vi "ValidateWSDL.vi"(8 "error in (no error)":errorcluster, 11 "WSDL URL":string) -> (0 "error out":errorcluster, 3 "WSDL URL (out)":string)   [LabVIEW 2017, in "WebServiceImporter.lvlib" / "ProxyDll Generator.lvlib"]
doc: "Download WSDL from given URL, validate WSDL content, ..."
uses:
  <vilib>/Platform/WebService/ProxyDll Generator/ProxyDll Generator.lvlib
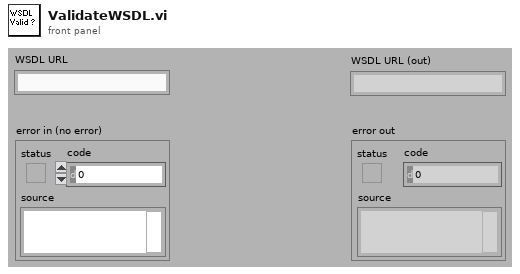
[diagram p1: front panel]
types:
  T1 = cluster{"Need Proxy":bool, "Username":string, "Password":string, "Domain":string, "Address":string, "Port":i32, "Need Authentication":bool}
  T2 = cluster{"Need Authentication":bool, "Username":string, "Password":string, "Domain":string}
  T3 = cluster{"Use Proxy Server":bool, "Address":string, "Port":u32}
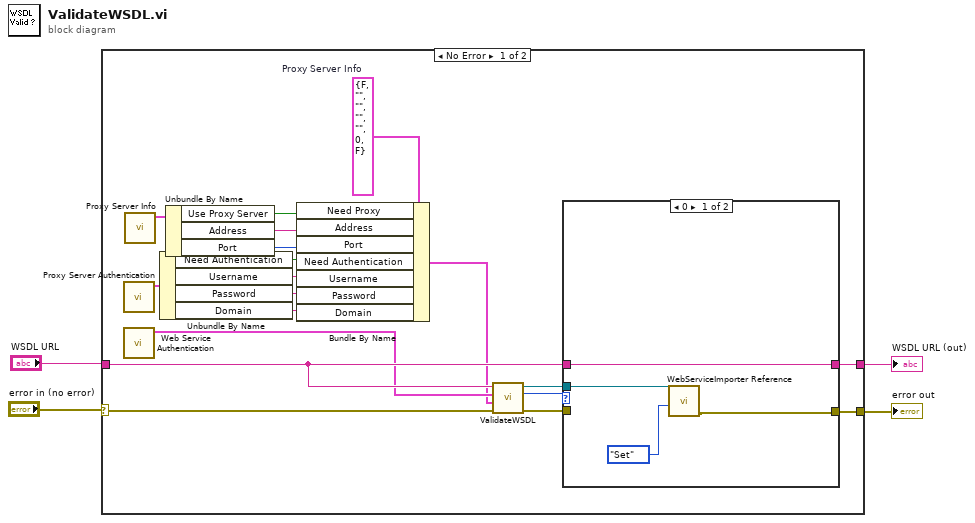
[diagram p0: block diagram]
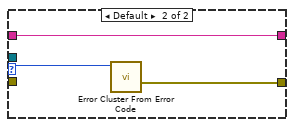
[diagram p2: hidden frame]
diagram:
  n1 = case shown="No Error" "error in (no error)" {
    selector: "error in (no error)" -> [w23 w32]
    tunnel: [w21 w32] -> w4
    tunnel: "WSDL URL" -> [w20 w31]
    tunnel: [w19 w31] -> w1
    frame No Error {
      w6 = T1 {"Need Proxy"=FALSE, "Username"="", "Password"="", "Domain"="", "Address"="", "Port"=0, "Need Authentication"=FALSE}  # Proxy Server Info
      n2 = call <vilib>:"Proxy Server Authentication.vi"() -> ("Web Service Authentication 2"=w11:T2)  [unwired: 10 in, 1 out]
      n3 = call <vilib>:"Web Service Authentication.vi"() -> ("Web Service Authentication 2"=w16:T2)  [unwired: 10 in, 1 out]
      n4 = call <vilib>:"Proxy Server Info.vi"() -> ("Proxy Server Info 2"=w15:T3)  [unwired: 10 in, 1 out]
      n5 = Unbundle By Name(w11) -> ("Need Authentication"=w10:bool, "Username"=w9:string, "Password"=w8:string, "Domain"=w7:string)
      n6 = Unbundle By Name(w15) -> ("Use Proxy Server"=w14:bool, "Address"=w13:string, "Port"=w12:u32)
      n7 = Bundle By Name(cluster=w6, "Need Proxy"=w14, "Address"=w13, "Port"=w12, "Need Authentication"=w10, "Username"=w9, "Password"=w8, "Domain"=w7) -> (w5:T1)
      n8 = call <vilib>:"ValidateWSDL.vi"("error in (no error)"=w23, "Proxy Server Info"=w5, "Web Service Authentication"=w16, "URL in"=w20) -> ("error out"=w17:errorcluster, "ErrorCode"=w18:i32, "Web Service Importer Ref"=w22:refnum<k24>)  [unwired: 5 in]
      n9 = case shown="0" w18 {
        selector: w18 -> [_ w28]
        tunnel: w22 -> [w26 _]
        tunnel: [w24 w30] -> w21
        tunnel: w20 -> [w25 w29]
        tunnel: [w25 w29] -> w19
        tunnel: w17 -> [_ _]
        frame 0 {
          n10 = call <vilib>:"WebServiceImporter Reference.vi"("Operation"=enum16{"Get", "Set"}."Set", "Web Service Importer"=w26) -> ("error out"=w24:errorcluster)  [unwired: 8 in, 1 out]
        }
        frame Default {
          n11 = call <vilib>:"Error Cluster From Error Code.vi"("error code (0)"=w28) -> ("error out"=w30:errorcluster)  [unwired: 8 in]
        }
      }
    }
    frame Error {
    }
  }
  "error out" <- w4
  "WSDL URL (out)" <- w1
